vi "Auto scripting split autonmous modes from text.vi"(11 "String":string) -> (2 "Programs":string[](array[string]), 3 "Program Name":string[](array[string]))   [LabVIEW 2013]
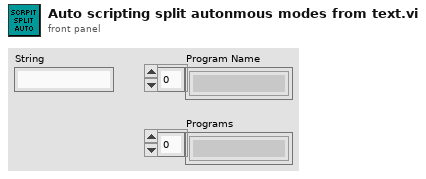
[diagram p1: front panel]
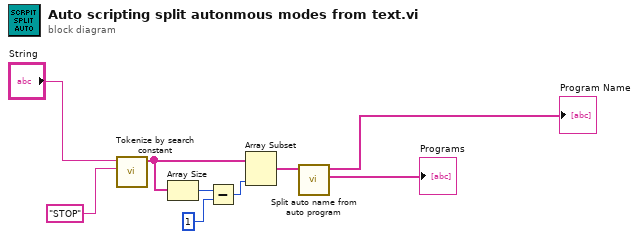
[diagram p0: block diagram]
diagram:
  n1 = call "Tokenize by search constant.vi"("search constant"="STOP", "Data"="String") -> ("Array"=w4:string[])  [unwired: 9 in]
  n2 = Array Size(array=w4) -> (size(s)=w5:i32)
  n3 = Subtract(x=w5, y=1) -> (x-y=w6:i32)
  n4 = Array Subset(array=w4, length=w6) -> (w3:string[])  [unwired: 1 in]
  n5 = call "Split auto name from auto program.vi"("Programs with names"=w3) -> ("Programs"=→"Programs":string[], "Program Name"=→"Program Name":string[])  [unwired: 9 in]
